vi "Klimageraet Ansteuerung.vi"(8 "Service aktiv":bool, 10 "Einschalten ab":sgl, 11 "Schaltschranktemperatur":sgl) -> (3 "Klimagerät EIN":bool)   [LabVIEW 2020, in "Allgemein.lvlib"]
uses:
  Allgemein.lvlib
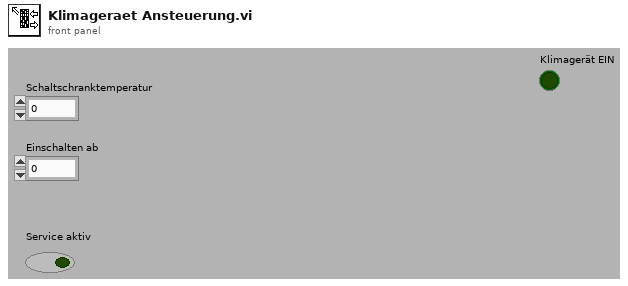
[diagram p1: front panel]
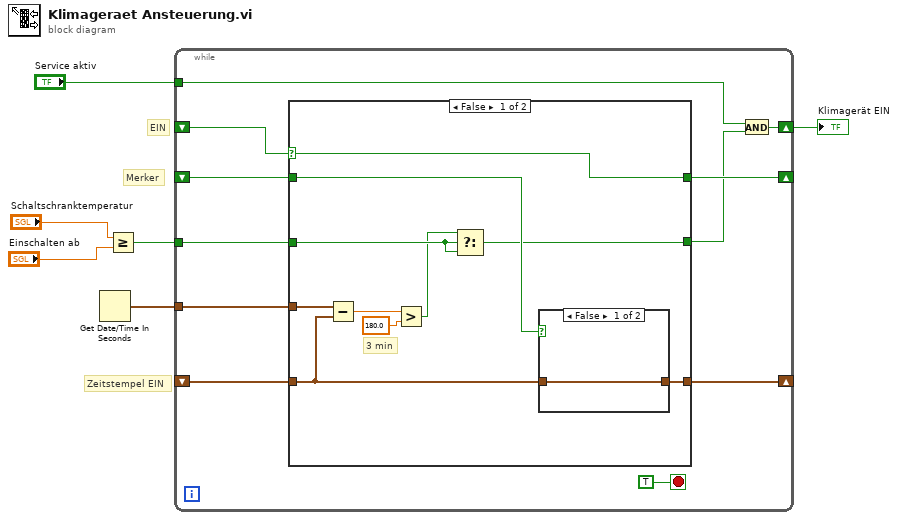
[diagram p0: block diagram]
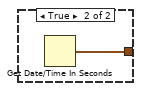
[diagram p2: hidden frame]
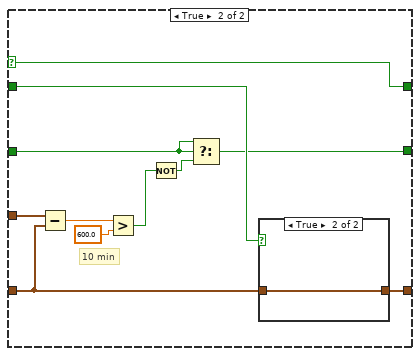
[diagram p3: hidden frame]
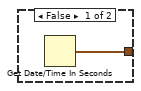
[diagram p4: hidden frame]
diagram:
  # "Merker"
  # "Zeitstempel EIN"
  # "EIN"
  n1 = Get Date/Time In Seconds() -> (seconds since 1Jan1904=w2:timestamp)
  n2 = Greater Or Equal?(x="Schaltschranktemperatur", y="Einschalten ab") -> (x >= y?=w4:bool)
  n3 = while {
    shift-right: [w9] -> w1
    shift-left: _ -> [w11]
    tunnel: w4 -> [w7]
    tunnel: "Service aktiv" -> [w8]
    shift-right: [w16] -> _
    shift-left: _ -> [w13]
    tunnel: w2 -> [w12]
    shift-right: [w14] -> _
    shift-left: _ -> [w15]
    stop <- TRUE stop-if-true
    n4 = case shown="False" w11 {
      selector: w11 -> [w22 w35]
      tunnel: [w27 w40] -> w16
      tunnel: w15 -> [w21 w34]
      tunnel: [w22 w35] -> w14
      tunnel: w13 -> [w24 w37]
      tunnel: w7 -> [w20 w33]
      tunnel: w12 -> [w23 w36]
      tunnel: [w18 w30] -> w10
      frame False {
        # "3 min"
        n5 = Subtract(x=w23, y=w24) -> (x-y=w26:dbl)
        n6 = Greater?(x=w26, y=180.0) -> (0:w19:bool)
        n7 = Select(t=w19, s=w20, f=w20) -> (s? t:f=w18:bool)
        n8 = case shown="False" w21 {
          tunnel: [w28 w29] -> w27
          tunnel: w24 -> [w28 _]
          frame False {
          }
          frame True {
            n9 = Get Date/Time In Seconds() -> (seconds since 1Jan1904=w29:timestamp)
          }
        }
      }
      frame True {
        # "10 min"
        n10 = Subtract(x=w36, y=w37) -> (x-y=w39:dbl)
        n11 = Greater?(x=w39, y=600.0) -> (0:w31:bool)
        n12 = Not(x=w31) -> (.not. x?=w32:bool)
        n13 = Select(t=w33, s=w33, f=w32) -> (s? t:f=w30:bool)
        n14 = case shown="True" w34 {
          tunnel: [w41 w42] -> w40
          tunnel: w37 -> [_ w42]
          frame False {
            n15 = Get Date/Time In Seconds() -> (seconds since 1Jan1904=w41:timestamp)
          }
          frame True {
          }
        }
      }
    }
    n16 = And(x=w8, y=w10) -> (x .and. y?=w9:bool)
  }
  "Klimagerät EIN" <- w1
